vi "UHR-Fleezers Control (host) - 11.9c.vi"() -> ()   [LabVIEW 2014] (continued)
                  }
                }
                n3318 = case shown="True" w5167 {
                  tunnel: w5226 -> [w5258 w5270]
                  tunnel: [w5258 w5262] -> w5222
                  tunnel: "Save ave N" -> [_ w5263]
                  tunnel: w5217 -> [_ w5261]
                  frame False {
                  }
                  frame True {
                    n3319 = Array Size(array=w5270) -> (size(s)=w5264:i32)
                    n3320 = Array Size(array=w5261) -> (size(s)=w5260:i32)
                    n3321 = Divide(x=w5264, y=w5260) -> (x/y=w5268:dbl)
                    n3322 = Reshape Array(w5270, w5268, w5260) -> (w5269:i16[][])
                    n3323 = Transpose 2D Array(2D array=w5269) -> (transposed array=w5267:i16[][])
                    n3324 = for {
                      tunnel: w5267 -> [w5273] mode=indexing
                      tunnel: [w5272] -> w5259 mode=indexing
                      tunnel: w5263 -> [w5271]
                      workers-P: _ -> [_]
                      n3325 = call "downsample 1D array - I16.vi"("Ave N"=w5271, "Array In"=w5273) -> ("Array Out"=w5272:i16[])  [unwired: 1 out]
                    }
                    n3326 = Transpose 2D Array(2D array=w5259) -> (transposed array=w5266:i16[][])
                    n3327 = Divide(x=w5264, y=w5263) -> (x/y=w5265:dbl)
                    n3328 = Reshape Array(w5266, w5265) -> (w5262:i16[])
                  }
                }
                n3329 = Index Array(array=w5188, index=1) -> (element=w5191:waveform(dbl))
                n3330 = Index Array(array=w5188, index=0) -> (element=w5193:waveform(dbl))
                n3331 = Unbundle By Name(w5191) -> ("Y"=w5195:dbl[])
                n3332 = Unbundle By Name(w5193) -> ("Y"=w5203:dbl[])
                n3333 = case "Write trap pos. data" shown="True" w5170 {
                  tunnel: w5169 -> [_ w5251]
                  tunnel: w5165 -> [_ w5250]
                  frame False {
                  }
                  frame True {
                    n3334 = Write to Binary File(file (use dialog)=w5251, data=w5250, 5:FALSE ("prepend array or string size? (T)"), 9:T25."big-endian, network order" ("byte order (0:big-endian, network order)")) -> ()  [unwired: 1 in, 4 out]
                  }
                }
                n3335 = Write to Binary File(file (use dialog)=w5229, data=w5222, 5:FALSE ("prepend array or string size? (T)"), 9:T25."big-endian, network order" ("byte order (0:big-endian, network order)")) -> ()  [unwired: 1 in, 4 out]
                n3336 = feedback #39(w5195) -> (w5197:dbl[])
                n3337 = Build Array (concatenate)(w5197, w5195) -> (w5196:dbl[])
                n3338 = Select(t=w5195, s=w5161, f=w5196) -> (s? t:f=w5181:dbl[])
                n3339 = feedback-in #39(w5181) -> ()
                n3340 = feedback #40(w5203) -> (w5216:dbl[])
                n3341 = Build Array (concatenate)(w5216, w5203) -> (w5215:dbl[])
                n3342 = Select(t=w5203, s=w5161, f=w5215) -> (s? t:f=w5190:dbl[])
                n3343 = feedback-in #40(w5190) -> ()
                n3344 = Divide(x=w5230, y=w5231) -> (x/y=w5233:dbl)
                n3345 = Multiply(x=w5233, y=100.0) -> (x*y=w5232:dbl)
                n3346 = Build Array(w5190, w5181) -> (→"Saved APD":dbl[][])
                n3347 = Array Size(array=w5190) -> (size(s)=w5208:i32)
                n3348 = Unbundle By Name(w5210) -> ("Y"=w5214:dbl[])
                n3349 = Subtract(x=w5208, y="N pts to average") -> (x-y=w5184:i32)
                n3350 = Multiply(x="N pts to average", y=u16 2) -> (x*y=w5185:u16)
                n3351 = Subtract(x=w5208, y=w5185) -> (x-y=w5183:i32)
                n3352 = feedback #41(w5214) -> (w5213:dbl[])
                n3353 = Build Array (concatenate)(w5213, w5214) -> (w5212:dbl[])
                n3354 = Select(t=w5214, s=w5161, f=w5212) -> (s? t:f=w5211:dbl[])
                "Trap Delta Graph" <- w5211
                n3355 = feedback-in #41(w5211) -> ()
                n3356 = Array Subset(array=w5190, index=w5184, length="N pts to average") -> (w5207:dbl[])
                n3357 = Array Subset(array=w5190, index=w5183, length="N pts to average") -> (w5206:dbl[])
                n3358 = Array Subset(array=w5181, index=w5184, length="N pts to average") -> (w5187:dbl[])
                n3359 = Array Subset(array=w5181, index=w5183, length="N pts to average") -> (w5186:dbl[])
                n3360 = Index Array(array=w5164, index=0) -> (element=w5162:waveform(dbl))
                n3361 = call-poly <vilib>:"Mean.vi"("X"=w5207) -> ("mean"=w5205:dbl)  [unwired: 1 out]
                n3362 = call-poly <vilib>:"Mean.vi"("X"=w5187) -> ("mean"=w5180:dbl)  [unwired: 1 out]
                n3363 = call-poly <vilib>:"Mean.vi"("X"=w5206) -> ("mean"=w5204:dbl)  [unwired: 1 out]
                n3364 = call-poly <vilib>:"Mean.vi"("X"=w5186) -> ("mean"=w5179:dbl)  [unwired: 1 out]
                n3365 = Unbundle By Name(w5162) -> ("Y"=w5159:dbl[])
                n3366 = Subtract(x=w5180, y=w5179) -> (x-y=w5171:dbl)
                "Delta Fl. 2" <- w5171
                n3367 = Subtract(x=w5205, y=w5204) -> (x-y=w5202:dbl)
                "Delta Fl. 1" <- w5202
                n3368 = Initialize Array(w5202, 1 ("dimension size")) -> (w5199:dbl[])
                n3369 = Initialize Array(w5171, 1 ("dimension size")) -> (w5176:dbl[])
                n3370 = feedback #42(w5199) -> (w5200:dbl[])
                n3371 = Build Array (concatenate)(w5200, w5199) -> (w5198:dbl[])
                n3372 = feedback #43(w5176) -> (w5177:dbl[])
                n3373 = Build Array (concatenate)(w5177, w5176) -> (w5175:dbl[])
                n3374 = feedback #44(w5159) -> (w5158:dbl[])
                n3375 = Build Array (concatenate)(w5158, w5159) -> (w5160:dbl[])
                n3376 = Select(t=w5159, s=w5161, f=w5160) -> (s? t:f=w5157:dbl[])
                "Saved trap pos" <- w5157
                n3377 = feedback-in #44(w5157) -> ()
                n3378 = Select(t=w5199, s=w5161, f=w5198) -> (s? t:f=w5174:dbl[])
                n3379 = feedback-in #42(w5174) -> ()
                n3380 = Select(t=w5176, s=w5161, f=w5175) -> (s? t:f=w5173:dbl[])
                n3381 = feedback-in #43(w5173) -> ()
                n3382 = Build Array(w5174, w5173) -> (→"Save APD Deriv":dbl[][])
              }
            }
            "Progress" <- w5140
            "Progress 2" <- w5140
          }
        }
      }
    }
    n3383 = Bundle By Name(cluster=w3733, "Green FB Ch 0"=w3732, "Green FB Ch 1"=w3731) -> (w3711:T49)
    "Green FB Signals (V)" <- w3711
    n3384 = Unbundle By Name(w3711) -> ("Green FB Ch 2"=→"Excitation laser intensities plot":dbl)
    n3385 = local read "wait to reset values"() -> (w3800:bool)
    n3386 = Not(x=w3798) -> (.not. x?=w3801:bool)
    n3387 = And(x=w3801, y=w3800) -> (x .and. y?=w3802:bool)
    n3388 = case "Part of MCL raster scanning: returns to initial positions after scan done" shown="True" w3802 {
      tunnel: w3520 -> [w4675 w4682]
      tunnel: [w4675 w4681] -> w3804
      tunnel: w3519 -> [w4674 w4680]
      tunnel: [w4674 w4679] -> w3799
      frame False {
      }
      frame True {
        w4690 = 10.0 ("y")
        w4689 = 32767.0 ("y")
        # "to return scan values\nafter a synchronous \nAOM scan"
        n3389 = local read "AO2"() -> (w4683:dbl)
        n3390 = local read "AO1"() -> (w4684:dbl)
        n3391 = local write "wait to reset values"(FALSE ("wait to reset values")) -> ()
        n3392 = Multiply(x=w4684, y=w4689) -> (x*y=w4686:dbl)
        n3393 = Multiply(x=w4683, y=w4689) -> (x*y=w4688:dbl)
        n3394 = Divide(x=w4686, y=w4690) -> (x/y=w4685:dbl)
        n3395 = Divide(x=w4688, y=w4690) -> (x/y=w4687:dbl)
        n3396 = To Word Integer(number=w4685) -> (16bit integer=w4691:i16)
        n3397 = To Word Integer(number=w4687) -> (16bit integer=w4692:i16)
        n3398 = local read "Total Counts (ticks)"() -> (w4676:u32)
        n3399 = xnode "Read/Write Control"("FPGA VI Reference In"=w4682, "error in"=w4680, "AO1"=w4691, "AO2"=w4692, "MCL count"=w4676) -> ("FPGA VI Reference Out"=w4681:T20, "error out"=w4679:errorcluster)
        n3400 = local read "Scan Range (V)\n(of steps)"() -> (w4677:dbl)
        n3401 = property on="Scan Range (V)\n(of steps)" class="DigNum (strict)"("Val(Sgnl)"=w4677) -> ()  [unwired: 2 in, 2 out]
      }
    }
    n3402 = node-c288() -> ()  [unwired: 2 out]
  }
  n3403 = VISA Close(VISA resource name=w111, error in (no error)=w110) -> (error out=w155:errorcluster)
  n3404 = call <vilib>:"Simple Error Handler.vi"("error in (no error)"=w155) -> ()  [unwired: 1 in, 8 out]
  n3405 = node-c288(w117) -> ()  [unwired: 1 out]
  n3406 = node-c288(w199) -> ()  [unwired: 1 out]
  n3407 = flat-sequence {
    tunnel: w291 -> [w5277]
    tunnel: w293 -> [w5278]
    tunnel: [w5276] -> w272
    tunnel: [w5275] -> w271
    tunnel: w255 -> [_]
    tunnel: w207 -> [_]
    tunnel: w123 -> [_]
    tunnel: w272 -> [w5279]
    tunnel: w271 -> [w5280]
    frame #0 {
      w5274 = FALSE ("AI to FIFO")
      n3408 = xnode "Read/Write Control"("FPGA VI Reference In"=w5278, "error in"=w5277, "AI to FIFO"=w5274, "APD to FIFO"=w5274) -> ("FPGA VI Reference Out"=w5276:T20, "error out"=w5275:errorcluster)
    }
    frame #1 {
      n3409 = xnode "Close FPGA VI Reference"("FPGA VI Reference In"=w5279, "error in"=w5280) -> ("error out"=→"error out":errorcluster)
    }
  }
